vi "ReadImageHeaderFile.vi"(1 "ImageHeaderFile":path=path "C:/AzCam/systems/mont4k/FitsTemplates/FitsTemplate_mont4k_green.txt") -> ()   [LabVIEW 2014]
doc: "Use this template to build a standard state machine design pattern. Each state executes code and determines which state to transition to. Contrast this design pattern with the user interface event pattern, in which code executes in response to user actions. Contrast this design pattern also with the queued message handler pattern, in which each message handling code can queue zero or more new messages."
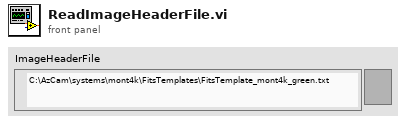
[diagram p1: front panel]
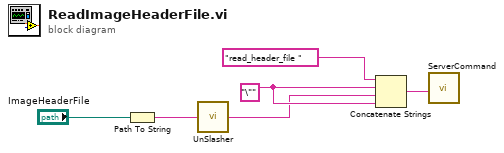
[diagram p0: block diagram]
diagram:
  w3 = "\""
  n1 = Path To String(path="ImageHeaderFile") -> (string=w2:string)
  n2 = call "UnSlasher.vi"("String In"=w2) -> ("String Out"=w1:string)
  n3 = Concatenate Strings("read_header_file " ("string"), w3, w1, w3) -> (w4:string)
  n4 = call "ServerCommand.vi"("Command"=w4) -> ()  [unwired: 2 out]
